vi "XML Get Actuation Chassis.vi"(11 "Actuation Network":T2) -> (0 "PID Parameters":T3[](array[typedef]), 1 "Actuation Chassis Names":string[](array[string]), 2 "Number of Correctors":i32, 3 "Actuation Variable Names":string[][](array[string]), 4 "Inverse PS Matrix Mapping":u32[][](array[numeric]), 5 "PS Parameters":T1[](array[typedef]), 6 "PS Matrix Mapping":cluster{u32[]}[](array[cluster]), 7 "Selected Correctors":u32[](array[numeric]))   [LabVIEW 2011, in "XML VIs.lvlib"]
doc: "Extracts the Actuation Network configuration data (ordered by chassis) and builds dedicated clusters for each configuration (ordered by response matrix column indexes).\nThe \"PS Matrix Mapping\" is used to decode the digital I/O of all Actuation Chassis to byte words representing each chasiss digital I/Os (each bit comes from one of the 8 chassis actuators) to a vector of boolean values in the response matrix column indexes order. \nThe \"Inverse PS Matrix Mapping\" is used to encode the digital I/O of all Actuation Chassis from a vector of boolean values in the response matrix column indexes order to byte words representing each chasiss digital I/Os (each bit comes from one of the 8 chassis actuators)."
uses:
  XML VIs.lvlib
  Types Definitions/Type PID Parameters.ctl
  Types Definitions/Type Actuation Network Configuration.ctl
  Types Definitions/Type PS Parameters.ctl
  Type Definitions.lvlib
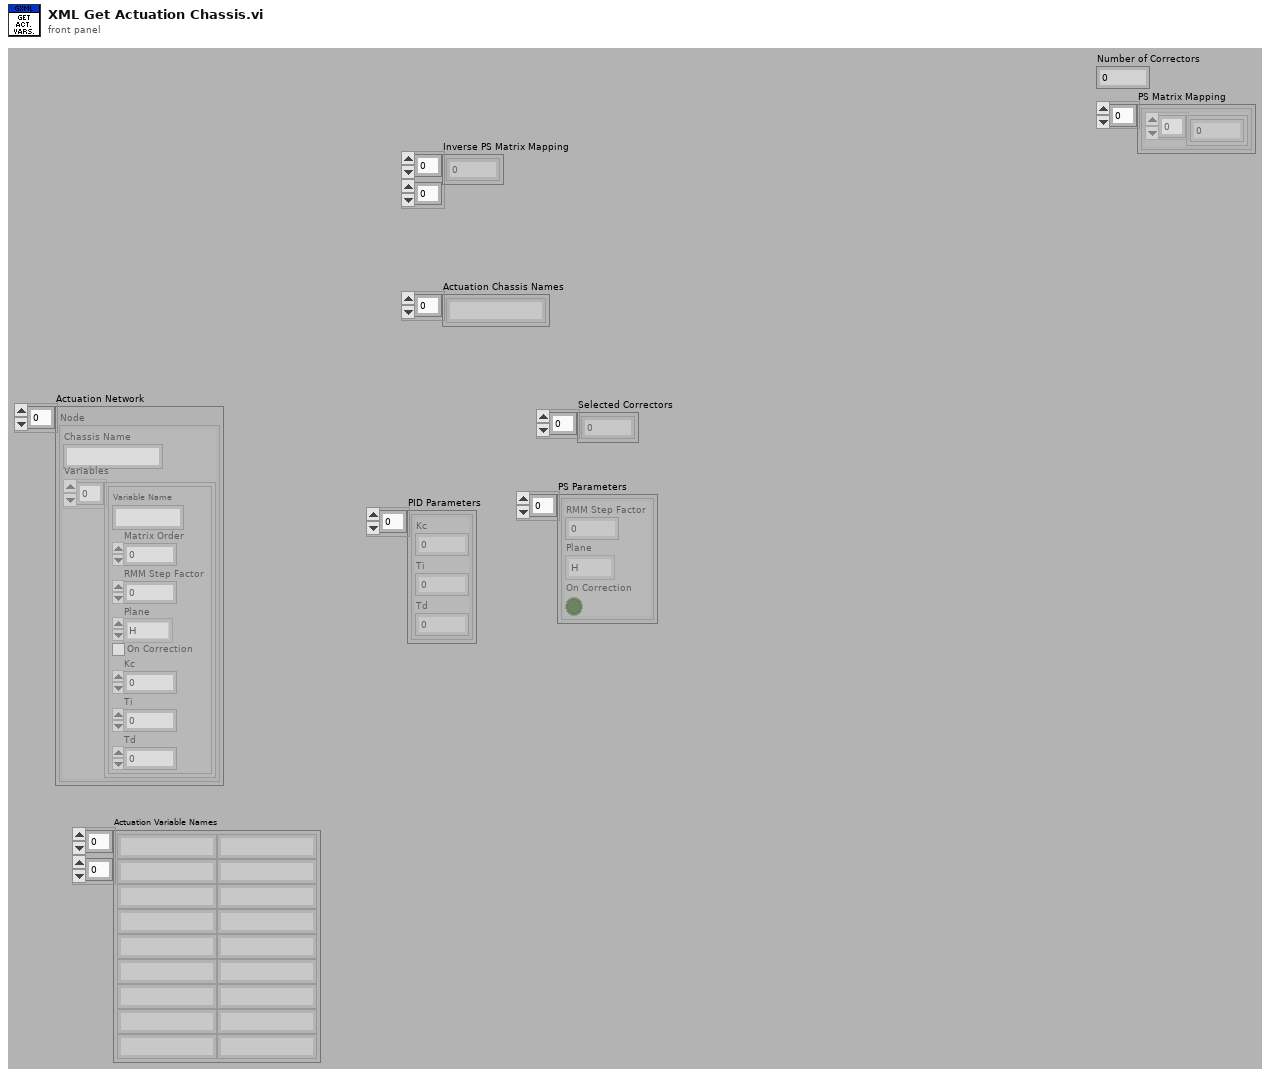
[diagram p1: front panel]
types:
  T1 = typedef "Type Definitions.lvlib/Type PS Parameters.ctl" = cluster{"RMM Step Factor":dbl, "Plane":enum8{"H", "V"}, "On Correction":bool}
  T2 = typedef "Type Definitions.lvlib/Type Actuation Network Configuration.ctl" = cluster{"Chassis Name":string, "Variables":cluster{"Variable Name":string, "Matrix Order":u32, "RMM Step Factor":dbl, "Plane":enum8{"H", "V"}, "On Correction":bool, "Kc":dbl, "Ti":dbl, "Td":dbl}[]}[]
  T3 = typedef "Type Definitions.lvlib/Type PID Parameters.ctl" = cluster{"Kc":fxp<+/-,16,8>, "Ti":fxp<+/-,16,8>, "Td":fxp<+/-,16,8>}
  T4 = cluster{"Variable Name":string, "Matrix Order":u32, "RMM Step Factor":dbl, "Plane":enum8{"H", "V"}, "On Correction":bool, "Kc":dbl, "Ti":dbl, "Td":dbl}[]
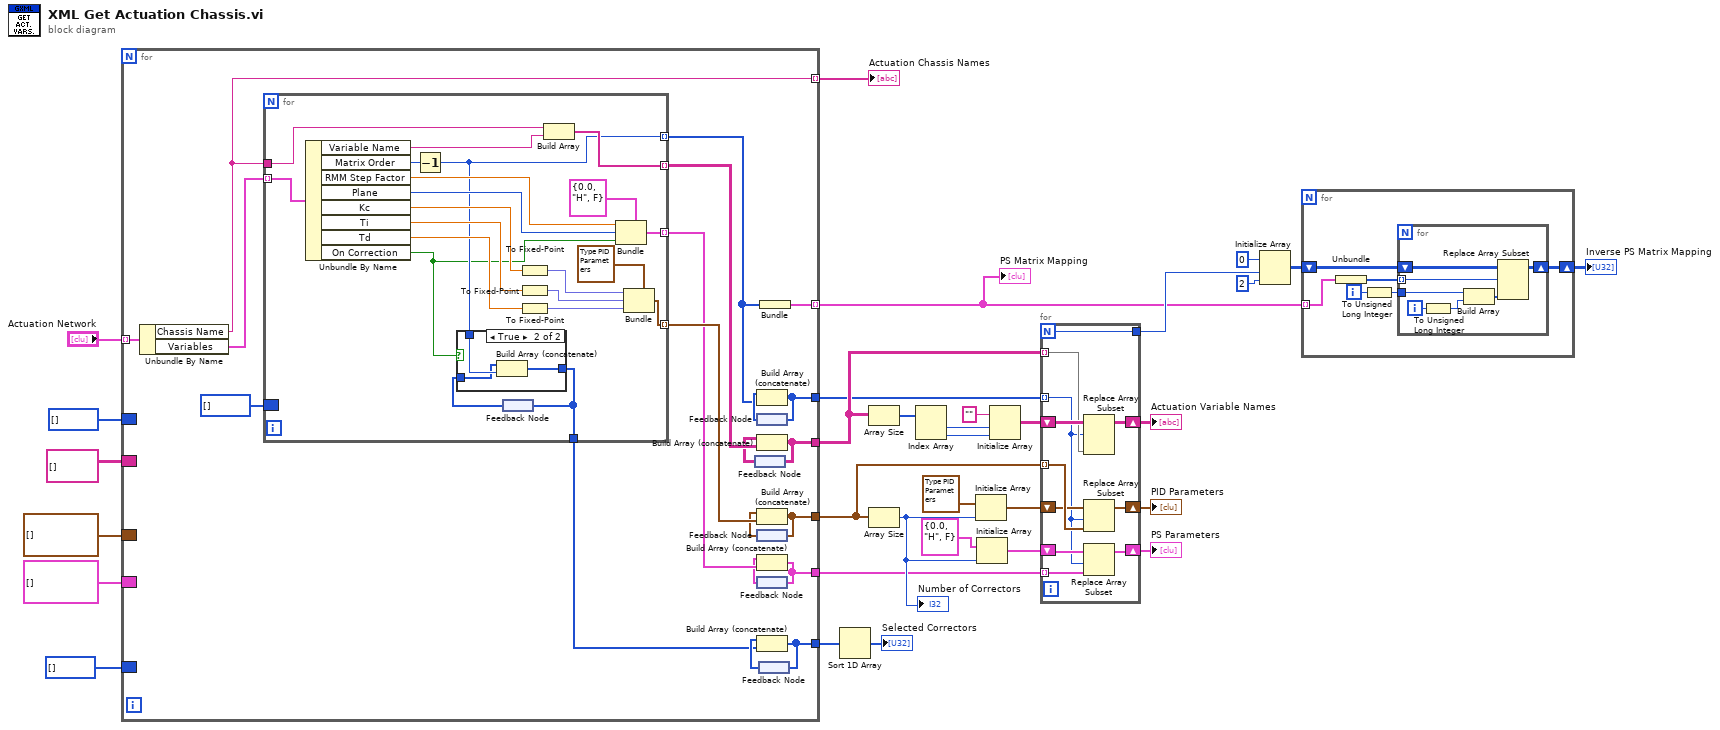
[diagram p0: block diagram]
diagram:
  n1 = for {
    tunnel: "Actuation Network" -> [w52] mode=indexing
    tunnel: [w45] -> w21 mode=indexing
    border: T1[] [] -> [_]
    tunnel: [w42] -> w8
    border: T3[] [] -> [_]
    tunnel: [w41] -> w7
    border: string[][] [] -> [_]
    tunnel: [w40] -> w6
    border: u32[] [] -> [_]
    tunnel: [w39] -> w5
    border: u32[] [] -> [_]
    tunnel: [w37] -> w3
    tunnel: [w33] -> w1 mode=indexing
    n2 = Unbundle By Name(w52) -> ("Chassis Name"=w45:string, "Variables"=w51:T4)
    n3 = for {
      tunnel: w51 -> [w73] mode=indexing
      tunnel: w45 -> [w71]
      tunnel: [w56] -> w34 mode=indexing
      tunnel: [w70] -> w50 mode=indexing
      tunnel: [w69] -> w47 mode=indexing
      tunnel: [w58] -> w44 mode=indexing
      border: u32[] [] -> [_]
      tunnel: [w54] -> w35
      n4 = Unbundle By Name(w73) -> ("Variable Name"=w72:string, "Matrix Order"=w64:u32, "RMM Step Factor"=w60:dbl, "Plane"=w59:enum8{"H", "V"}, "Kc"=w61:dbl, "Ti"=w62:dbl, "Td"=w63:dbl, "On Correction"=w53:bool)
      n5 = Decrement(x=w64) -> (x-1=w56:u32)
      n6 = feedback #1() -> (w55:u32[])
      n7 = case shown="True" w53 {
        tunnel: w56 -> [_ w77]
        tunnel: w55 -> [w74 w76]
        tunnel: [w74 w75] -> w54
        frame False {
        }
        frame True {
          n8 = Build Array (concatenate)(w76, w77) -> (w75:u32[])
        }
      }
      n9 = feedback-in #1(w54) -> ()
      n10 = To Fixed-Point(number=w61) -> (fixed-point=w67:fxp<+/-,16,8>)  [unwired: 1 in]
      n11 = To Fixed-Point(number=w62) -> (fixed-point=w68:fxp<+/-,16,8>)  [unwired: 1 in]
      n12 = To Fixed-Point(number=w63) -> (fixed-point=w66:fxp<+/-,16,8>)  [unwired: 1 in]
      n13 = Build Array(w71, w72) -> (w70:string[])
      n14 = Bundle(cluster=T1 {"RMM Step Factor"=0.0, "Plane"=enum."H", "On Correction"=FALSE}, "RMM Step Factor"=w60, "Plane"=w59, "On Correction"=w53) -> (w58:T1)
      n15 = Bundle(cluster=T3 {"Kc"=0.0, "Ti"=0.0, "Td"=0.0}, "Kc"=w67, "Ti"=w68, "Td"=w66) -> (w69:T3)
    }
    n16 = feedback #2() -> (w49:string[][])
    n17 = feedback #3() -> (w48:u32[])
    n18 = Build Array (concatenate)(w48, w34) -> (w39:u32[])
    n19 = feedback-in #3(w39) -> ()
    n20 = Build Array (concatenate)(w49, w50) -> (w40:string[][])
    n21 = feedback-in #2(w40) -> ()
    n22 = feedback #4() -> (w46:T3[])
    n23 = Build Array (concatenate)(w46, w47) -> (w41:T3[])
    n24 = feedback-in #4(w41) -> ()
    n25 = feedback #5() -> (w43:T1[])
    n26 = Build Array (concatenate)(w43, w44) -> (w42:T1[])
    n27 = feedback-in #5(w42) -> ()
    n28 = feedback #6() -> (w36:u32[])
    n29 = Build Array (concatenate)(w36, w35) -> (w37:u32[])
    n30 = feedback-in #6(w37) -> ()
    n31 = Bundle(w34) -> (w33:cluster{u32[]})  [unwired: 1 in]
  }
  "Actuation Chassis Names" <- w21
  "PS Matrix Mapping" <- w1
  n32 = Sort 1D Array(array=w3) -> (sorted array=→"Selected Correctors":u32[])
  n33 = Array Size(array=w6) -> (size(s)=w30:i32[])
  n34 = Array Size(array=w7) -> (size(s)=w13:i32)
  "Number of Correctors" <- w13
  n35 = Index Array(array=w30) -> (element #1=w29:i32, element #2=w28:i32)  [unwired: 2 in]
  n36 = Initialize Array(T3 {"Kc"=0.0, "Ti"=0.0, "Td"=0.0}, w13) -> (w24:T3[])
  n37 = Initialize Array(T1 {"RMM Step Factor"=0.0, "Plane"=enum."H", "On Correction"=FALSE} ("cluster"), w13) -> (w12:T1[])
  n38 = Initialize Array("" ("element"), w29, w28) -> (w27:string[][])
  n39 = for {
    N -> [w82]
    tunnel: w6 -> [w86] mode=indexing
    tunnel: w5 -> [w78] mode=indexing
    shift-right: [w87] -> w26
    shift-left: w27 -> [w88]
    tunnel: w7 -> [w85] mode=indexing
    shift-right: [w83] -> w23
    shift-left: w24 -> [w84]
    tunnel: [w82] -> w14
    tunnel: w8 -> [w79] mode=indexing
    shift-right: [w80] -> w9
    shift-left: w12 -> [w81]
    n40 = Replace Array Subset(array=w88, new element=w86, index (row)=w78) -> (w87:string[][])  [unwired: 1 in]
    n41 = Replace Array Subset(array=w84, new element=w85, index=w78) -> (w83:T3[])
    n42 = Replace Array Subset(array=w81, new element=w79, index=w78) -> (w80:T1[])
  }
  "Actuation Variable Names" <- w26
  "PID Parameters" <- w23
  "PS Parameters" <- w9
  n43 = Initialize Array(u32 0 ("element"), w14, 2 ("dimension size")) -> (w16:u32[][])
  n44 = for {
    shift-right: [w93] -> w15
    shift-left: w16 -> [w94]
    tunnel: w1 -> [w90] mode=indexing
    i -> [w92]
    n45 = Unbundle(w90) -> (w89:u32[])
    n46 = To Unsigned Long Integer(number=w92) -> (unsigned 32bit integer=w91:u32)
    n47 = for {
      tunnel: w91 -> [w99]
      shift-right: [w100] -> w93
      shift-left: w94 -> [w101]
      tunnel: w89 -> [w95] mode=indexing
      i -> [w96]
      n48 = To Unsigned Long Integer(number=w96) -> (unsigned 32bit integer=w97:u32)
      n49 = Build Array(w99, w97) -> (w98:u32[])
      n50 = Replace Array Subset(array=w101, new element=w98, index (row)=w95) -> (w100:u32[][])  [unwired: 1 in]
    }
  }
  "Inverse PS Matrix Mapping" <- w15
